vi "Configure Blender.vi"(4 "Trigger Event 4(\"\")":string, 5 "Trigger Event 3(\"\")":string, 6 "Trigger Event 2(\"\")":string, 7 "Trigger Event 1(\"\")":string, 8 "error in (no error)":errorcluster, 9 "Boolean Operation (1: AND)":i32(ring)=1 items=["OR", "AND"], 10 "Blender Number (1: Blender 1)":i32(ring)=1 items=["Blender 1"=1, "Blender 2"=2], 11 "VISA resource name":refnum<visa-resource-name>) -> (0 "error out":errorcluster, 3 "VISA resource name out":refnum<visa-resource-name>)   [LabVIEW 2023, in "Keithley DMM6500 DAQ6500 Series.lvlib"]
doc: "Selects whether the blender performs OR operations or AND operations, and specifies the events that trigger the blender"
uses:
  <instrlib>/Keithley DMM6500 DAQ6500 Series/Keithley DMM6500 DAQ6500 Series.lvlib
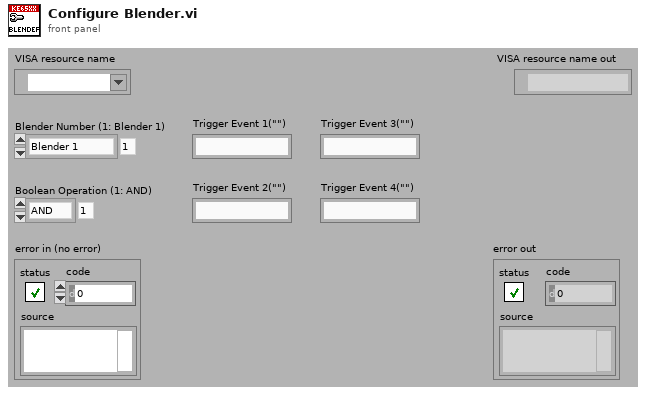
[diagram p1: front panel]
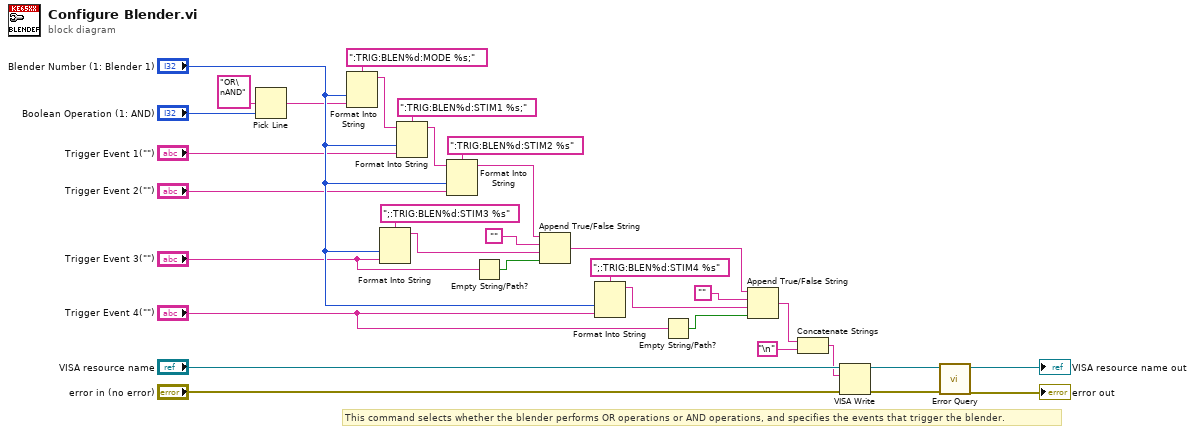
[diagram p0: block diagram]
diagram:
  # "This command selects whether the blender performs OR operations or AND operations, and specifies the events that trigger the blender."
  n1 = Pick Line(multi-line string="OR\nAND", line index="Boolean Operation (1: AND)") -> (output string=w28:string)  [unwired: 1 in]
  n2 = Format Into String(format string=":TRIG:BLEN%d:MODE %s;", "Blender Number (1: Blender 1)", w28) -> (resulting string=w27:string)  [unwired: 2 in, 1 out]
  n3 = Format Into String(format string=";:TRIG:BLEN%d:STIM3 %s", "Blender Number (1: Blender 1)", "Trigger Event 3(\"\")") -> (resulting string=w7:string)  [unwired: 2 in, 1 out]
  n4 = Format Into String(format string=":TRIG:BLEN%d:STIM1 %s;", initial string=w27, "Blender Number (1: Blender 1)", "Trigger Event 1(\"\")") -> (resulting string=w24:string)  [unwired: 1 in, 1 out]
  n5 = Format Into String(format string=":TRIG:BLEN%d:STIM2 %s", initial string=w24, "Blender Number (1: Blender 1)", "Trigger Event 2(\"\")") -> (resulting string=w11:string)  [unwired: 1 in, 1 out]
  n6 = Empty String/Path?(string/path="Trigger Event 3(\"\")") -> (empty?=w6:bool)
  n7 = Append True/False String(1:w6, 2:w7, 3:"", 4:w11) -> (0:w10:string)
  n8 = Format Into String(format string=";:TRIG:BLEN%d:STIM4 %s", "Blender Number (1: Blender 1)", "Trigger Event 4(\"\")") -> (resulting string=w4:string)  [unwired: 2 in, 1 out]
  n9 = Empty String/Path?(string/path="Trigger Event 4(\"\")") -> (empty?=w2:bool)
  n10 = Append True/False String(1:w2, 2:w4, 3:"", 4:w10) -> (0:w9:string)
  n11 = Concatenate Strings(w9, "\n") -> (w13:string)
  n12 = VISA Write(VISA resource name="VISA resource name", write buffer=w13, error in (no error)="error in (no error)") -> (VISA resource name out=w18:refnum<visa-resource-name>, error out=w17:errorcluster)  [unwired: 1 out]
  n13 = call <instrlib>:"Error Query.vi"("error in (no error)"=w17, "VISA resource name"=w18) -> ("error out"=→"error out":errorcluster, "VISA resource name out"=→"VISA resource name out":refnum<visa-resource-name>)  [unwired: 6 in, 2 out]
